vi "kernal_smooth.vi"(11 "array":i16[](array[numeric])) -> (3 "Array":i16[](array[numeric]))   [LabVIEW 2012]
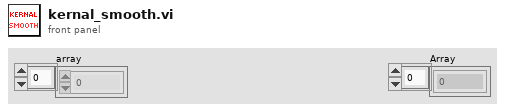
[diagram p1: front panel]
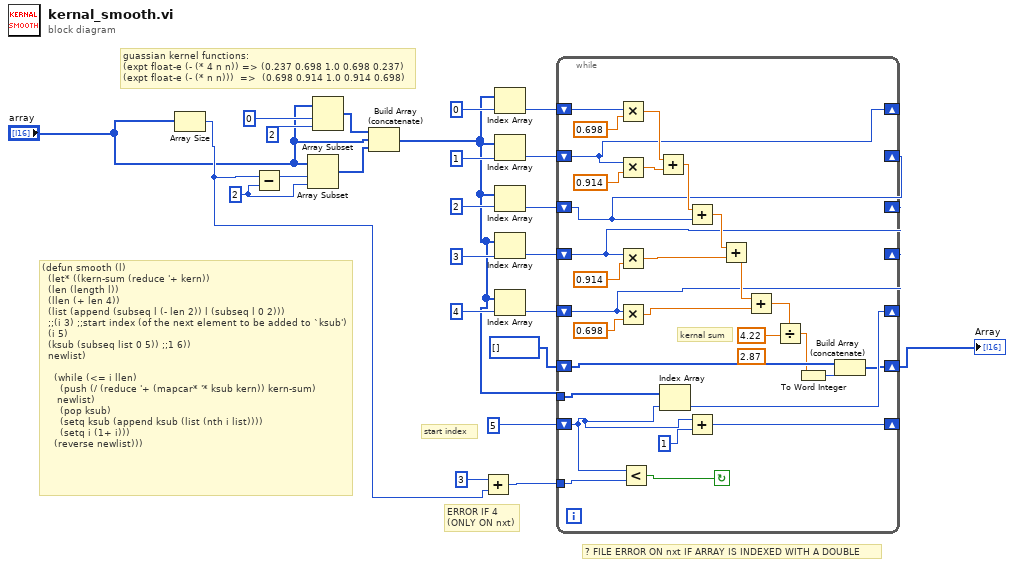
[diagram p0: block diagram]
diagram:
  w22 = i16 2 ("x")
  # "ERROR IF 4\n(ONLY ON nxt)"
  # "? FILE ERROR ON nxt IF ARRAY IS INDEXED WITH A DOUBLE"
  # "guassian kernel functions:\n(expt float-e (- (* 4 n n)) => (0.237 0.698 1.0 0.698 0.237)\n(expt float-e (- (* n n)))  =>  (0.698 0.914 1.0 0.914 0.698)"
  # "start index"
  # "(defun smooth (l)\n  (let* ((kern-sum (reduce '+ kern))\n\t (len (length l))\n\t (llen (+ len 4))\n\t (list (append (subseq l (- len 2)) l (subseq l 0 2)))\n\t ;;(i 3) ;;start index (of the next element to be added to `ksub')\n\t (i 5)\n\t (ksub (subseq list 0 5)) ;;1 6)) \n\t newlist)\n\t\n    (while (<= i llen) \n      (push (/ (reduce '+ (mapcar* '* ksub kern)) kern-sum)\n\t    newlist)\n      (pop ksub)\n      (setq ksub (append ksub (list (nth i list))))\n      (setq i (1+ i)))\n    (reverse newlist)))"
  n1 = Array Size(array="array") -> (size(s)=w16:i32)
  n2 = Subtract(x=w16, y=w22) -> (x-y=w23:i32)
  n3 = Array Subset(array="array", index=w23, length=w22) -> (w18:i16[])
  n4 = Array Subset(array="array", index=i16 0 ("x"), length=i16 2 ("x")) -> (w19:i16[])
  n5 = Build Array (concatenate)(w19, "array", w18) -> (w4:i16[])
  n6 = Add(x=i16 3, y=w16) -> (x+y=w15:i32)
  n7 = Index Array(array=w4, index=i16 0 ("x")) -> (element=w14:i16)
  n8 = Index Array(array=w4, index=i16 1 ("x")) -> (element=w9:i16)
  n9 = Index Array(array=w4, index=i16 2 ("x")) -> (element=w8:i16)
  n10 = Index Array(array=w4, index=i16 3 ("x")) -> (element=w7:i16)
  n11 = Index Array(array=w4, index=i16 4 ("x")) -> (element=w6:i16)
  n12 = while {
    shift-right: [w36] -> _
    shift-left: i16 5 ("x") -> [w25]
    tunnel: w15 -> [w53]
    shift-right: [w31] -> _
    shift-left: w14 -> [w52]
    shift-right: [w32] -> _
    shift-left: w9 -> [w31]
    shift-right: [w33] -> _
    shift-left: w8 -> [w32]
    shift-right: [w34] -> _
    shift-left: w7 -> [w33]
    shift-right: [w35] -> _
    shift-left: w6 -> [w34]
    tunnel: w4 -> [w47]
    shift-right: [w29] -> w2
    shift-left: i16[] [] -> [w30]
    stop <- w26 continue-if-true
    (unwired) 2.87
    # "kernal sum"
    n13 = Multiply(x=w52, y=0.698) -> (x*y=w45:dbl)
    n14 = Multiply(x=w31, y=0.914) -> (x*y=w46:dbl)
    n15 = Multiply(x=w33, y=0.914) -> (x*y=w42:dbl)
    n16 = Multiply(x=w34, y=0.698) -> (x*y=w40:dbl)
    n17 = Less?(x=w25, y=w53) -> (x < y?=w26:bool)
    n18 = Add(x=w45, y=w46) -> (x+y=w44:dbl)
    n19 = Index Array(array=w47, index=w25) -> (element=w35:i16)
    n20 = Add(x=w44, y=w32) -> (x+y=w43:dbl)
    n21 = Add(x=w25, y=i16 1 ("x")) -> (x+y=w36:i16)
    n22 = Add(x=w43, y=w42) -> (x+y=w41:dbl)
    n23 = Add(x=w41, y=w40) -> (x+y=w39:dbl)
    n24 = Divide(x=w39, y=4.22) -> (x/y=w27:dbl)
    n25 = To Word Integer(number=w27) -> (16bit integer=w28:i16)
    n26 = Build Array (concatenate)(w30, w28) -> (w29:i16[])
  }
  "Array" <- w2
